vi "httpc.vi"(8 "error in (no error)":errorcluster, 9 "index":i32, 10 "ITFileSave path":path, 11 "Data_in":T1) -> (0 "error out":errorcluster, 3 "Data_out":T1)   [LabVIEW 2014]
uses:
  controls/Data1.ctl
  controls/Payjson.ctl
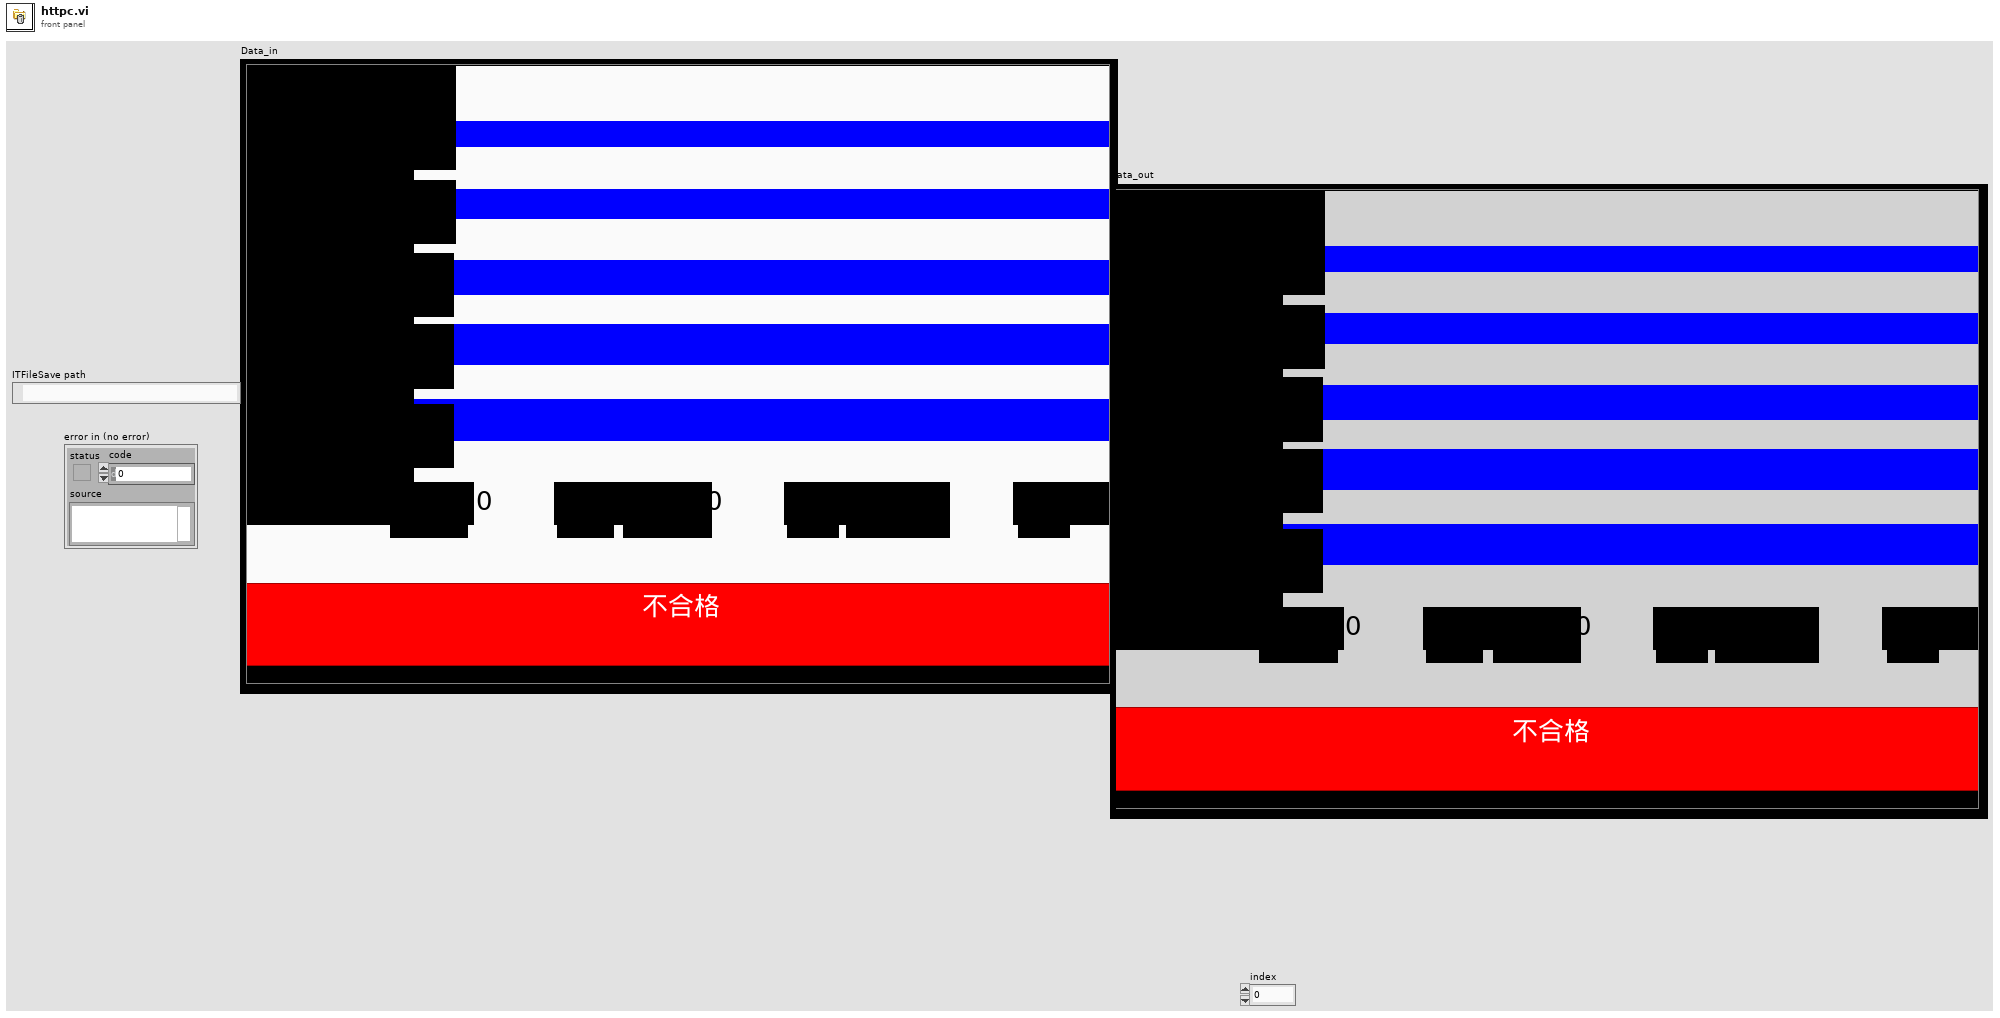
[diagram p1: front panel]
types:
  T1 = typedef "Data1.ctl" = cluster{"Date":string, "BarCode1":string, "BarCode2":string, "BarCode3":string, "Message":string, "OK Count":u16, "NG Count":u16, "Total Count":u16, "ModelData":string[][], "OK&NG":bool, "COM1":refnum<visa-resource-name>, "COM2":refnum<visa-resource-name>, "IO":i32, "Time":u32, "TCP":refnum<k5>, "TCP 2":refnum<k5>, "COM1 2":refnum<visa-resource-name>, "CheckNum":string, "BarCode1_1":string, "BarCode2_1":string, "BarCode3_1":string, "日期":string, "機種":string, "機號":string, "商品條碼1":string, "OK_1":string, "OK":string, "NG":string, "NG_1":string, "Total":string, "Total_1":string, "ClaerTime":u32, "Pjson":T2, "LotNo":string[], "CheckParsArray":string[], "BarCode4":string, "BarCode4_1":string, "商品條碼2":string, "BarCode5":string, "BarCode5_1":string, "商品條碼3":string, "ReScanNG":i32, "NGTimeCT":u32}
  T2 = typedef "Payjson.ctl" = cluster{"DEPT":string, "LINE":string, "STANO":string, "WORKNO":string, "PRODSN":string, "COMPNTID":string, "COMPNTLOT":string, "COMPNTSN":string, "USEDQTY":i16, "OPDATE":string, "OPUSER":string, "RECVDATE":string, "MMODU":string}[]
  T3 = cluster{"DEPT":string, "LINE":string, "STANO":string, "WORKNO":string, "PRODSN":string, "COMPNTID":string, "COMPNTLOT":string, "COMPNTSN":string, "USEDQTY":i16, "OPDATE":string, "OPUSER":string, "RECVDATE":string, "MMODU":string}
  T4 = cluster{"DEPT":string, "LINE":string, "STANO":string, "WORKNO":string, "PRODSN":string, "COMPNTID":string, "COMPNTLOT":string, "COMPNTSN":string, "USEDQTY":i16, "OPDATE":string, "OPUSER":string, "RECVDATE":string, "MMODU":string}[]
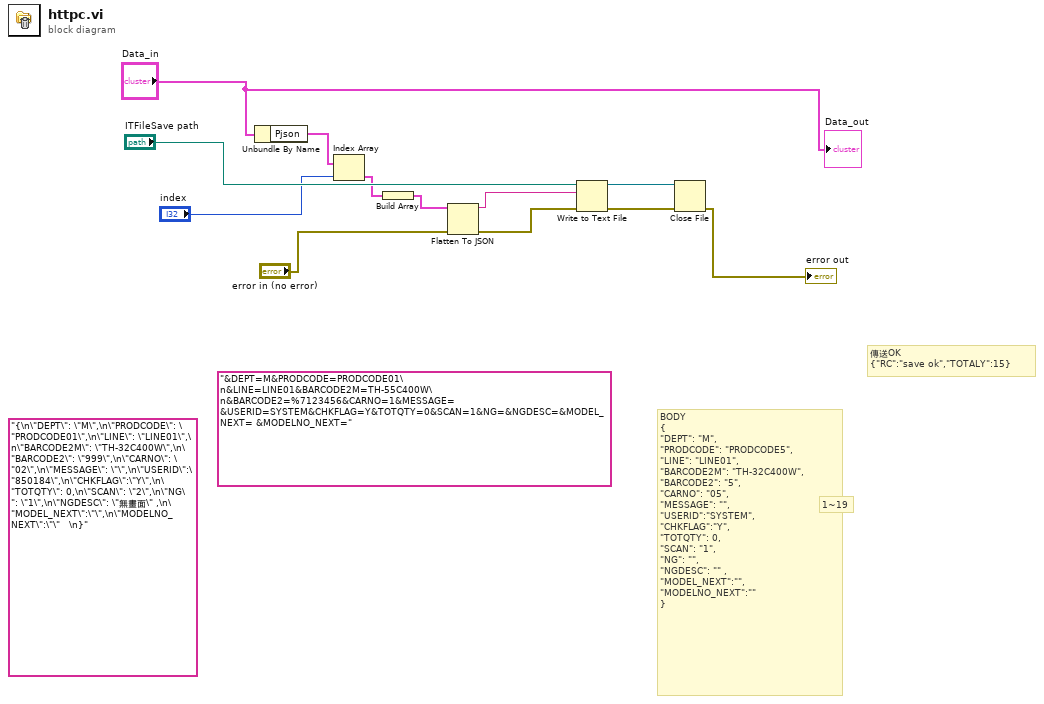
[diagram p0: block diagram]
diagram:
  (unwired) "&DEPT=M&PRODCODE=PRODCODE01\n&LINE=LINE01&BARCODE2M=TH-55C400W\n&BARCODE2=%7123456&CARNO=1&MESSAGE= &USERID=SYSTEM&CHKFLAG=Y&TOTQTY=0&SCAN=1&NG=&NGDESC=&MODEL_NEXT= &MODELNO_NEXT="
  (unwired) "{\n\"DEPT\": \"M\",\n\"PRODCODE\": \"PRODCODE01\",\n\"LINE\": \"LINE01\",\n\"BARCODE2M\": \"TH-32C400W\",\n\"BARCODE2\": \"999\",\n\"CARNO\": \"02\",\n\"MESSAGE\": \"\",\n\"USERID\":\"850184\",\n\"CHKFLAG\":\"Y\",\n\"TOTQTY\": 0,\n\"SCAN\": \"2\",\n\"NG\": \"1\",\n\"NGDESC\": \"無畫面\" ,\n\"MODEL_NEXT\":\"\",\n\"MODELNO_NEXT\":\"\"   \n}" ("buffer")
  # "傳送OK\n{\"RC\":\"save ok\",\"TOTALY\":15}"
  # "BODY\n{\n\"DEPT\": \"M\",\n\"PRODCODE\": \"PRODCODE5\",\n\"LINE\": \"LINE01\",\n\"BARCODE2M\": \"TH-32C400W\",\n\"BARCODE2\": \"5\",\n\"CARNO\": \"05\",\n\"MESSAGE\": \"\",\n\"USERID\":\"SYSTEM\",\n\"CHKFLAG\":\"Y\",\n\"TOTQTY\": 0,\n\"SCAN\": \"1\",\n\"NG\": \"\",\n\"NGDESC\": \"\" ,\n\"MODEL_NEXT\":\"\",\n\"MODELNO_NEXT\":\"\" \n}"
  # "1~19"
  n1 = Unbundle By Name("Data_in") -> ("Pjson"=w4:T2)
  n2 = Index Array(array=w4, index="index") -> (element=w3:T3)
  n3 = Build Array(w3) -> (w2:T4)
  n4 = Flatten To JSON(anything=w2, error in (no error)="error in (no error)") -> (JSON string=w11:string, 11:w8:errorcluster)  [unwired: 1 in]
  n5 = Write to Text File(file (use dialog)="ITFileSave path", text=w11, error in=w8) -> (refnum out=w10:refnum<file>, error out=w9:errorcluster)  [unwired: 1 in, 1 out]
  n6 = Close File(refnum=w10, error in=w9) -> (error out=→"error out":errorcluster)  [unwired: 1 out]
  "Data_out" <- "Data_in"
